vi "Teleop.vi"(10 "Match Info":T1={"Autonomous Elapsed Seconds"=0.0, "TeleOp Elapsed Seconds"=0.0, "Disabled Elapsed Seconds"=0.0, "Visited Autonomous"=FALSE, "Visited TeleOp"=FALSE, "Visited Disabled"=FALSE, "Autonomous Settings"={"Autonomous Style"=enum."Independent", "VI Refnum"=refnum}}, 11 "Call Context":T2) -> ()   [LabVIEW 2020]
doc: "This VI is called for each TeleOp packet received from the DS where the robot is not disabled. It is often used to read from the joysticks and update I/O or to update setpoints for timed control loops. It should complete and return within 20 milliseconds or it may miss DS packets."
uses:
  <vilib>/Rock Robotics/WPI/DriverStation/WPI_DriverStationDerivedRobotMode.ctl
  <vilib>/Rock Robotics/WPI/DriverStation/WPI_DriverStationMatch Info.ctl
  <vilib>/Rock Robotics/WPI/Solenoid/WPI_SolenoidValue.ctl
  <vilib>/Rock Robotics/WPI/ThirdParty/Phoenix-LabVIEW/Motor Controller/Controls/CTRE_Phoenix_MotorControl_ControlMode.ctl
  <vilib>/Rock Robotics/WPI/Utilities/WPI_GetSetVariantRefNum.vi
  <vilib>/Rock Robotics/Network Tables/NT Write Numeric Array.vi
  <vilib>/Rock Robotics/Network Tables/NT Read Boolean.vi
  <vilib>/Rock Robotics/Network Tables/NT Read Number.vi
  <vilib>/Rock Robotics/WPI/Solenoid/Deprecated/WPI_SolenoidSetBool.vi
  Robot Global Data.vi
  <vilib>/Rock Robotics/WPI/Solenoid/WPI_SolenoidSetEnum.vi
  <vilib>/Rock Robotics/Network Tables/NT Write Number.vi
  <vilib>/Rock Robotics/Network Tables/NT Write Boolean Array.vi
  <vilib>/Rock Robotics/WPI/Solenoid/Deprecated/WPI_SolenoidGetBool.vi
panel:
  out "TargetValid 5":bool
  out "TargetValid 4":bool
  out "POVs":i16[](array[numeric])
  out "Sample Slider 0":dbl(slide) scale=0.0..5.0
  out "Sample Boolean 1":bool
  out "Sample Boolean 0":bool
  # "April tags"
  # "Retroreflective tape"
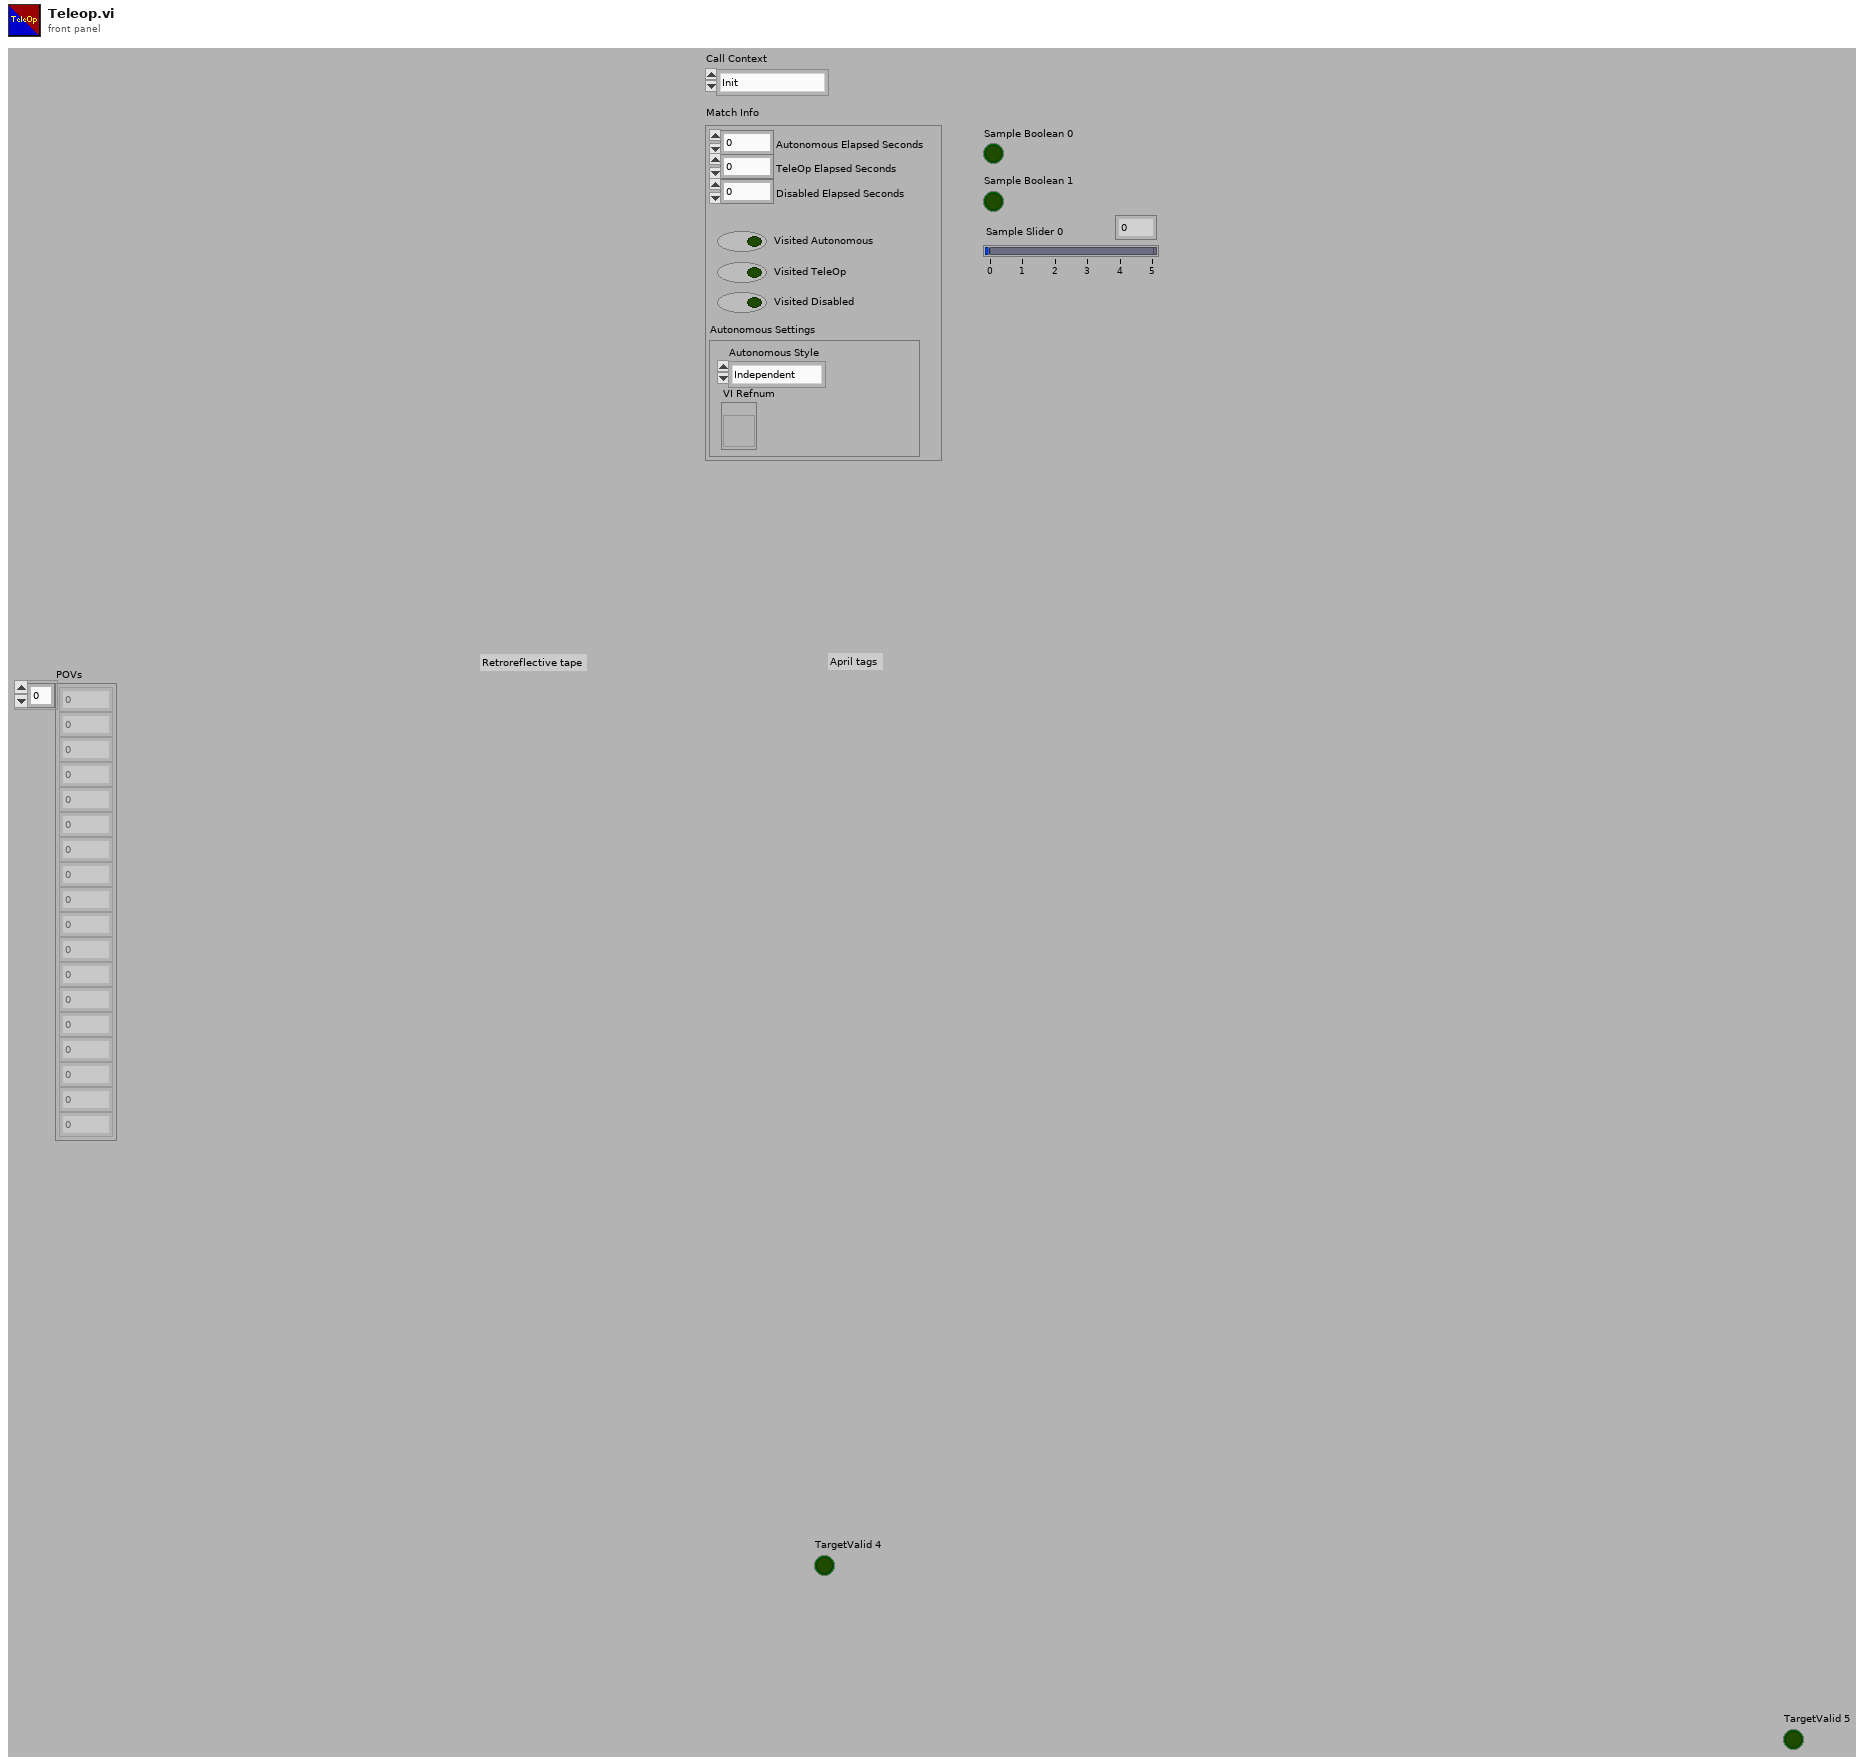
[diagram p1: front panel]
types:
  T1 = typedef "WPI_DriverStationMatch Info.ctl" = cluster{"Autonomous Elapsed Seconds":dbl, "TeleOp Elapsed Seconds":dbl, "Disabled Elapsed Seconds":dbl, "Visited Autonomous":bool, "Visited TeleOp":bool, "Visited Disabled":bool, "Autonomous Settings":cluster{"Autonomous Style":enum16{"Iterative", "Independent"}, "VI Refnum":refnum<vi>}}
  T2 = typedef "WPI_DriverStationDerivedRobotMode.ctl" = enum16{"Init", "Execute", "Stop"}
  T3 = typedef "WPI_SolenoidValue.ctl" = enum16{"Off", "On", "Forward", "Reverse"}
  T4 = cluster{"offsetAngle H":dbl, "offsetAngle V":dbl, "area":dbl, "skew":dbl}
  T5 = typedef "WPI_RobotDriveDevRef.ctl" = cluster{"DevStatus":errorcluster, "Motors[]":T6[], "Square Inputs":bool, "Max Output":dbl}
  T6 = typedef "WPI_MotorControlDeviceRef.ctl" = cluster{"DeviceStatus":errorcluster, "Type":T7, "PWM":cluster{"PWM Channel":T8, "DeadBand":T9}, "CAN":cluster{"Device Number":u8, "SetOutput VI Ref":variant, "GetOutput VI Ref":variant, "Enable VI Ref":variant, "Disable VI Ref":variant, "Data":variant}, "Invert":bool, "DIO PWM":cluster{"PWM \"Enable\" Channel":T8, "DIOChannel":T10, "PWM Rate":dbl}}
  T7 = typedef "WPI_MotorControlType.ctl" = enum16{"PWM", "CAN", "DIO PWM"}
  T8 = typedef "FPGA_DIOPWMChannel.ctl" = enum8{"PWM 0", "PWM 1", "PWM 2", "PWM 3", "PWM 4", "PWM 5", "PWM 6", "PWM 7", "PWM 8", "PWM 9", "PWM MXP 0", "PWM MXP 1", "PWM MXP 2", "PWM MXP 3", "PWM MXP 4", "PWM MXP 5", "PWM MXP 6", "PWM MXP 7", "PWM MXP 8", "PWM MXP 9", "Invalid"}
  T9 = typedef "WPI_PWMDeadband.ctl" = cluster{"Name":string, "maxPositivePwm":i32, "minPositivePwm":i32, "centerPwm":i32, "maxNegativePwm":i32, "minNegativePwm":i32, "angularRange":u16}
  T10 = typedef "FPGA_DIOChannel.ctl" = enum8{"DIO 0", "DIO 1", "DIO 2", "DIO 3", "DIO 4", "DIO 5", "DIO 6", "DIO 7", "DIO 8", "DIO 9", "DIO MXP 0", "DIO MXP 1", "DIO MXP 2", "DIO MXP 3", "DIO MXP 4", "DIO MXP 5", "DIO MXP 6", "DIO MXP 7", "DIO MXP 8", "DIO MXP 9", "DIO MXP 10", "DIO MXP 11", "DIO MXP 12", "DIO MXP 13", "DIO MXP 14", "DIO MXP 15", "SPI Port CS1", "SPI Port CS2", "SPI Port CS3", "SPI Port MISO", "SPI Port MOSI", "Invalid"}
  T11 = typedef "WPI_JoystickDevRef.ctl" = cluster{"Device":T12}
  T12 = typedef "WPI_JoystickDeviceEnum.ctl" = enum16{"USB 0", "USB 1", "USB 2", "USB 3", "USB 4", "USB 5"}
  T13 = cluster{"Buttons[0]":bool, "Buttons[1]":bool, "Buttons[2]":bool, "Buttons[3]":bool, "Buttons[4]":bool, "Buttons[5]":bool, "Buttons[6]":bool, "Buttons[7]":bool, "Buttons[8]":bool}
  T14 = cluster{"Axes[0]":dbl, "Axes[1]":dbl, "Axes[2]":dbl, "Axes[3]":dbl, "Axes[4]":dbl, "Axes[5]":dbl, "Axes[6]":dbl, "Axes[7]":dbl, "Axes[8]":dbl}
  T15 = typedef "WPI_SolenoidDevRef.ctl" = cluster{"DevStatus":errorcluster, "Pneumatics Control Module":u8, "Forward Solenoid Channel":T16, "Reverse Solenoid Channel":T16}
  T16 = typedef "WPI_SolenoidChannel.ctl" = enum8{"Solenoid 0", "Solenoid 1", "Solenoid 2", "Solenoid 3", "Solenoid 4", "Solenoid 5", "Solenoid 6", "Solenoid 7", "Solenoid 8", "Solenoid 9", "Solenoid 10", "Solenoid 11", "Solenoid 12", "Solenoid 13", "Solenoid 14", "Solenoid 15", "Invalid"}
  T17 = typedef "CTRE_Phoenix_MotorControl_ControlMode.ctl" = u16
  T18 = cluster{"Motors[][0]":T6, "Motors[][1]":T6, "Motors[][2]":T6, "Motors[][3]":T6, "Motors[][4]":T6, "Motors[][5]":T6, "Motors[][6]":T6, "Motors[][7]":T6, "Motors[][8]":T6}
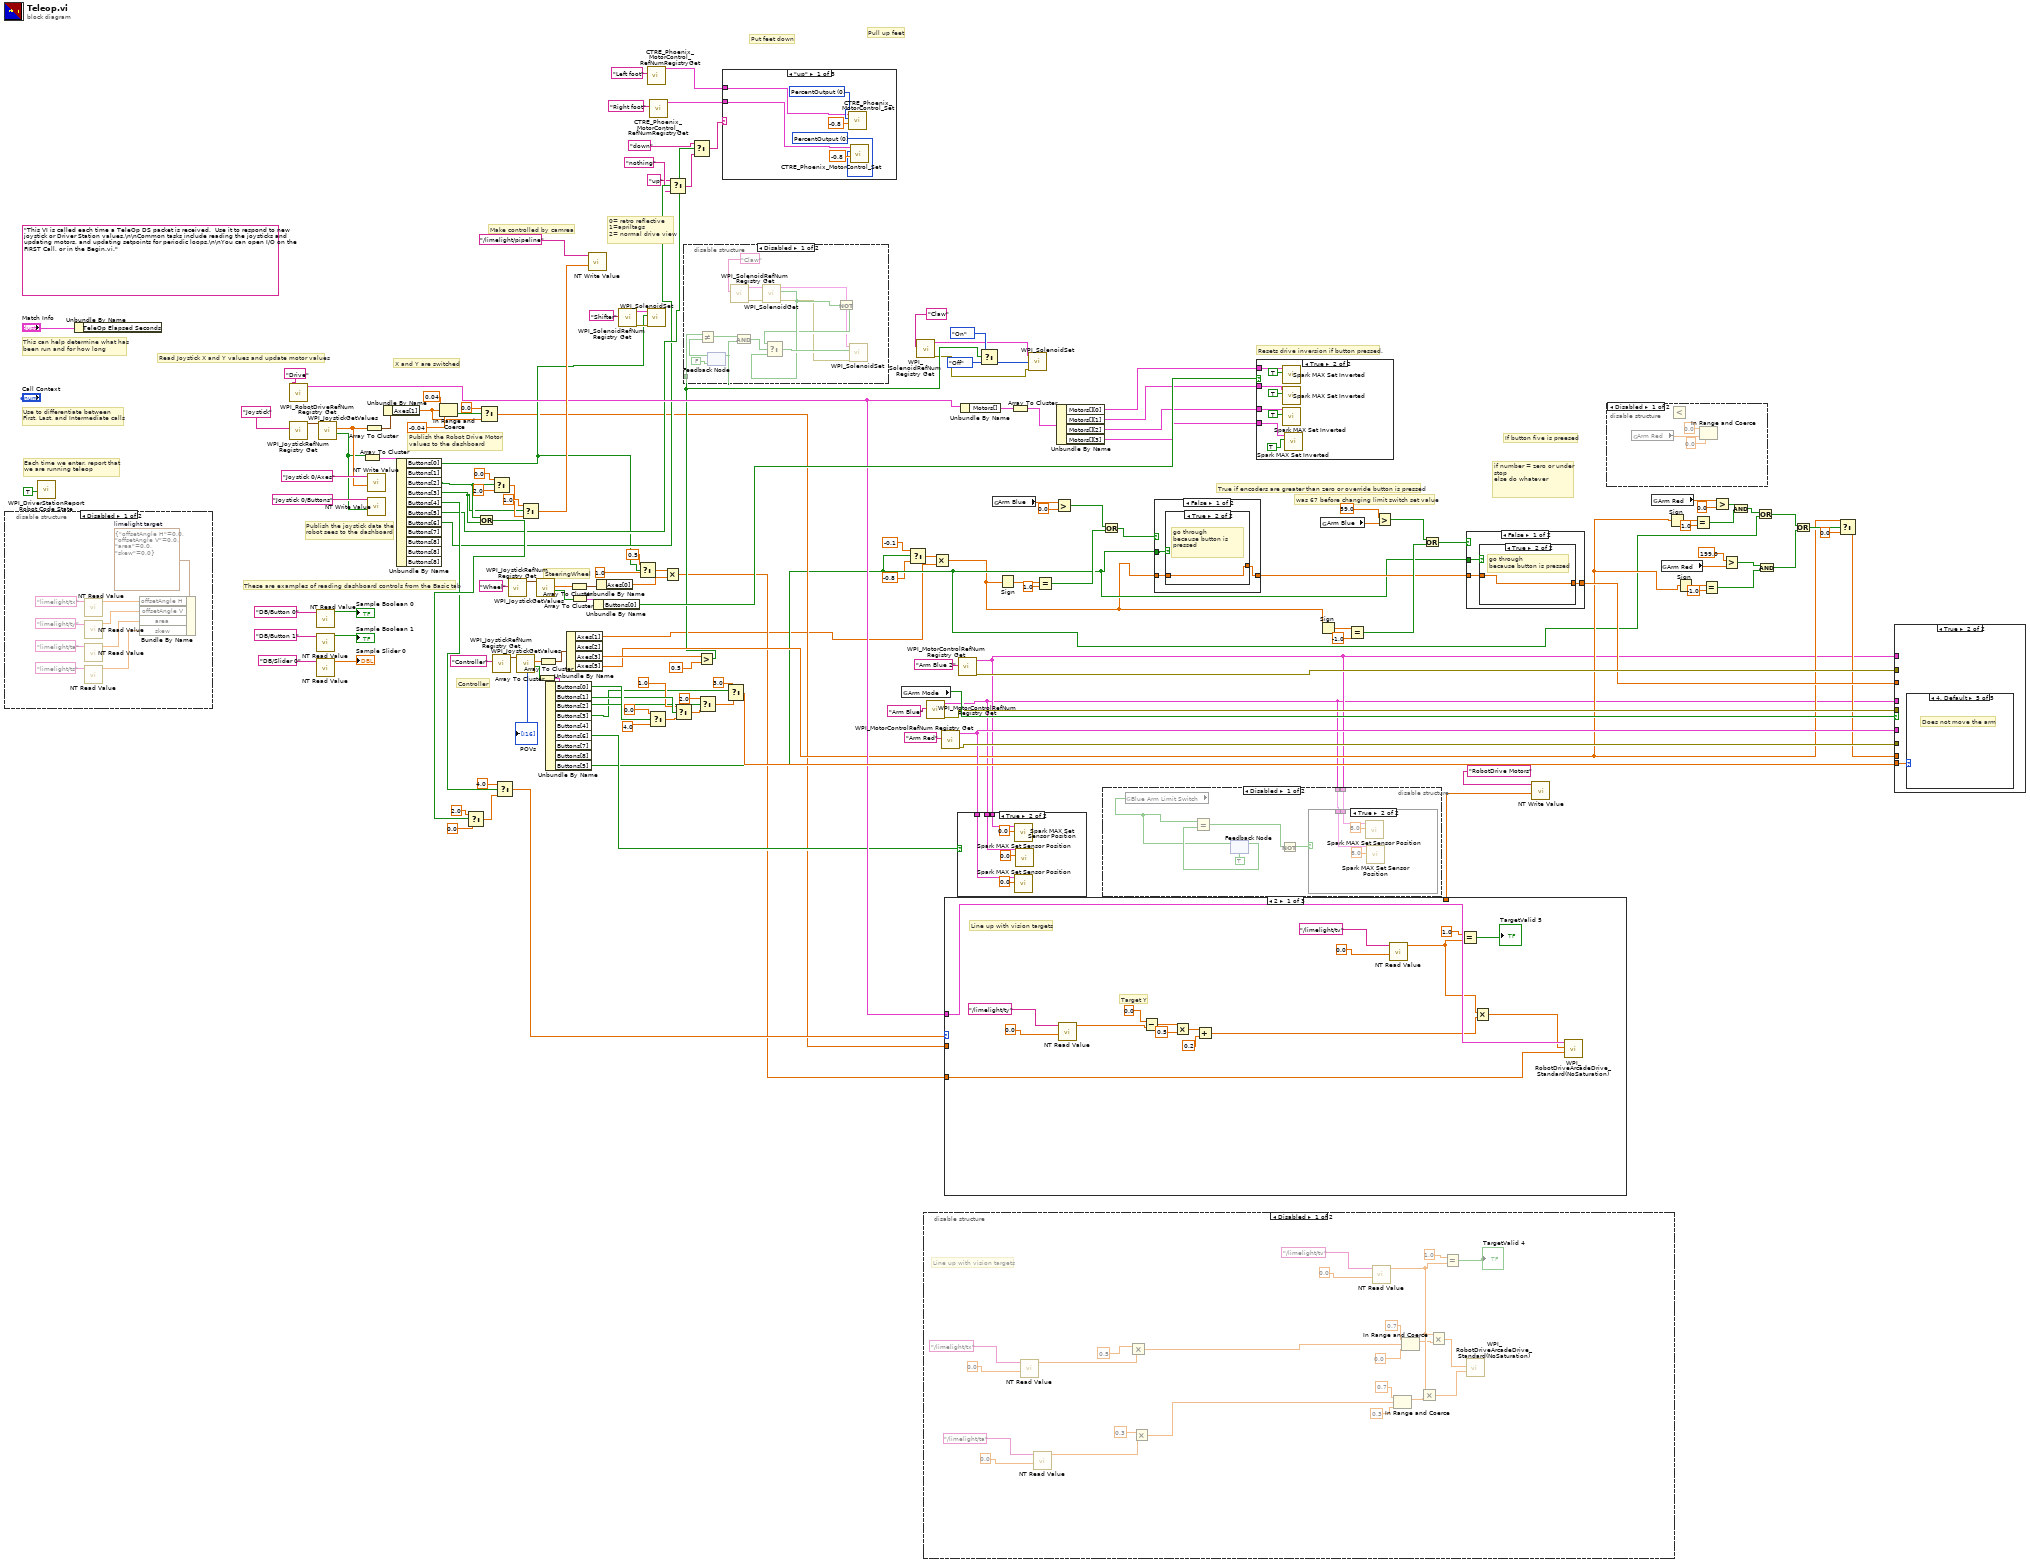
[diagram p0: block diagram]
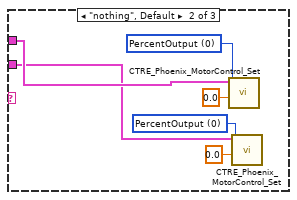
[diagram p6: hidden frame]
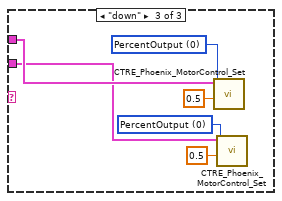
[diagram p7: hidden frame]
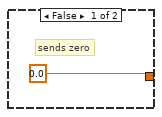
[diagram p8: hidden frame]
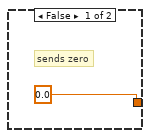
[diagram p10: hidden frame]
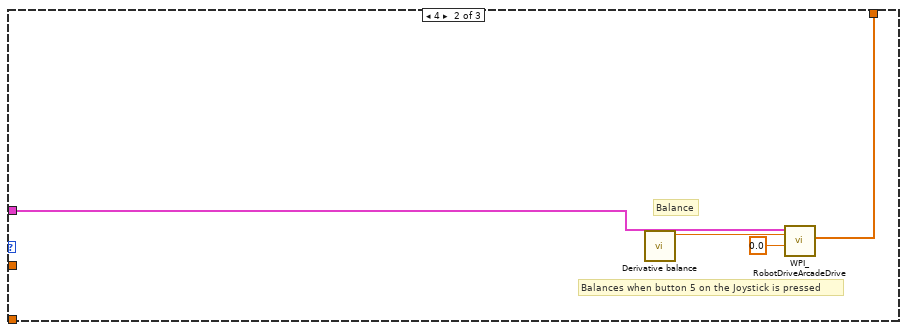
[diagram p15: hidden frame]
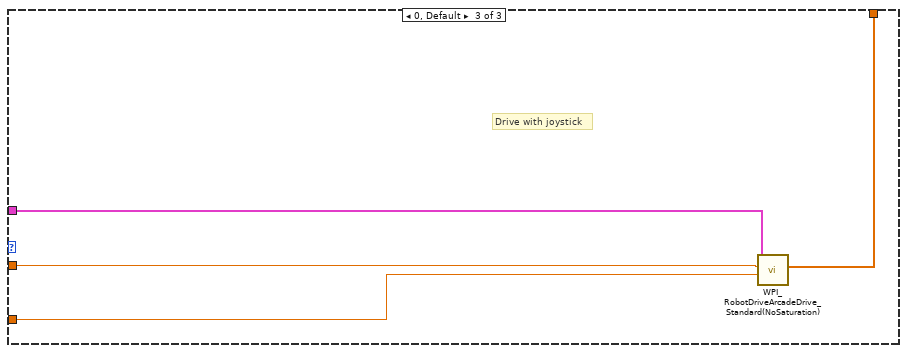
[diagram p16: hidden frame]
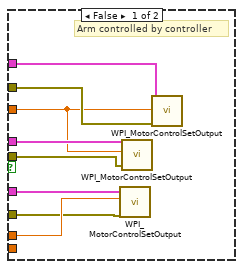
[diagram p17: hidden frame]
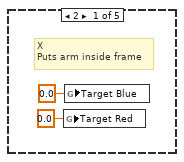
[diagram p18: hidden frame]
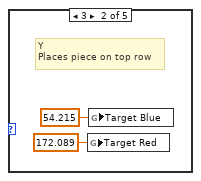
[diagram p19: hidden frame]
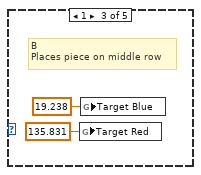
[diagram p20: hidden frame]
diagram:
  (unwired) "This VI is called each time a TeleOp DS packet is received.  Use it to respond to new joystick or Driver Station values.\n\nCommon tasks include reading the joysticks and updating motors, and updating setpoints for periodic loops.\n\nYou can open I/O on the FIRST Call, or in the Begin.vi."
  # "X and Y are switched"
  # "Put feet down"
  # "Pull up feet"
  # "was 67 before changing limit switch set value"
  # "True if encoders are greater than zero or override button is pressed"
  # "if number = zero or under\nstop\nelse do whatever"
  # "If button five is preesed"
  # "Resets drive inversion if button pressed."
  # "0= retro reflective\n1=apriltags\n2= normal drive view"
  # "Make controlled by camrea"
  # "SteeringWheel"
  # "Controller"
  # "These are examples of reading dashboard controls from the Basic tab"
  # "Publish the Robot Drive Motor\nvalues to the dashboard"
  # "Publish the joystick data the\nrobot sees to the dashboard"
  # "Each time we enter, report that\nwe are running teleop"
  # "Use to differentiate between\nFirst, Last, and Intermediate calls"
  # "This can help determine what has\nbeen run and for how long"
  # "Read Joystick X and Y values and update motor values"
  n1 = disable-structure shown="Disabled" {
    frame Disabled {
      w160 = T4 {"offsetAngle H"=0.0, "offsetAngle V"=0.0, "area"=0.0, "skew"=0.0}  # limelight target
      n2 = call-poly <vilib>:"NT Read Value.vi"("name"="limelight/tx" ("Name")) -> ("value"=w159:dbl)  [unwired: 8 in, 2 out]
      n3 = call-poly <vilib>:"NT Read Value.vi"("name"="limelight/ty" ("Name")) -> ("value"=w158:dbl)  [unwired: 8 in, 2 out]
      n4 = call-poly <vilib>:"NT Read Value.vi"("name"="limelight/ta" ("Name")) -> ("value"=w157:dbl)  [unwired: 8 in, 2 out]
      n5 = call-poly <vilib>:"NT Read Value.vi"("name"="limelight/ts" ("Name")) -> ("value"=w156:dbl)  [unwired: 8 in, 2 out]
      n6 = Bundle By Name(cluster=w160, "offsetAngle H"=w159, "offsetAngle V"=w158, "area"=w157, "skew"=w156) -> ()  [unwired: 1 out]
    }
    frame Enabled {
    }
  }
  n7 = call <vilib>:"WPI_DriverStationReport Robot Code State.vi"("TeleOp"=TRUE ("Autonomous")) -> ()  [unwired: 10 in, 1 out]
  n8 = Unbundle By Name("Match Info") -> ()  [unwired: 1 out]
  n9 = call <vilib>:"WPI_RobotDriveRefNum Registry Get.vi"("refnum name"="Drive") -> ("RobotDriveDevRef"=w80:T5)  [unwired: 1 in, 9 out]
  n10 = call <vilib>:"WPI_JoystickRefNum Registry Get.vi"("refnum name"="Joystick") -> ("JoystickDevRef"=w152:T11)  [unwired: 1 in, 9 out]
  n11 = call-poly <vilib>:"NT Read Value.vi"("name"="DB/Button 0" ("refnum name")) -> ("value"=→"Sample Boolean 0":bool)  [unwired: 8 in, 2 out]
  n12 = call-poly <vilib>:"NT Read Value.vi"("name"="DB/Slider 0" ("refnum name")) -> ("value"=→"Sample Slider 0":dbl)  [unwired: 8 in, 2 out]
  n13 = call-poly <vilib>:"NT Read Value.vi"("name"="DB/Button 1" ("refnum name")) -> ("value"=→"Sample Boolean 1":bool)  [unwired: 8 in, 2 out]
  n14 = call <vilib>:"WPI_JoystickGetValues.vi"("JoystickDevRef"=w152) -> ("Buttons"=w110:bool[], "Axes"=w141:dbl[])  [unwired: 6 in, 3 out]
  n15 = Array To Cluster(array=w110) -> (cluster=w109:T13)
  n16 = Array To Cluster(array=w141) -> (cluster=w140:T14)
  n17 = call-poly <vilib>:"NT Write Value.vi"("value"=w141, "name"="Joystick 0/Axes" ("Name")) -> ()  [unwired: 9 in, 1 out]
  n18 = call-poly <vilib>:"NT Write Value.vi"("value"=w110, "name"="Joystick 0/Buttons" ("Name")) -> ()  [unwired: 9 in, 1 out]
  n19 = Unbundle By Name(w140) -> ("Axes[1]"=w8:dbl)
  n20 = Unbundle By Name(w109) -> ("Buttons[0]"=w17:bool, "Buttons[2]"=w93:bool, "Buttons[3]"=w92:bool, "Buttons[4]"=w37:bool, "Buttons[5]"=w36:bool, "Buttons[6]"=w32:bool)  [unwired: 5 out]
  n21 = In Range and Coerce(upper limit=0.04, x=w8, lower limit=-0.04) -> (In Range?=w12:bool)  [unwired: 1 out]
  n22 = Or(x=w93, y=w92) -> (x .or. y?=w91:bool)
  n23 = Select(t=2.0, s=w91, f=0.0) -> (s? t:f=w106:dbl)
  n24 = Select(t=0.0, s=w12, f=w8) -> (s? t:f=w7:dbl)
  n25 = Select(t=0.0, s=w93, f=2.0) -> (s? t:f=w94:dbl)
  n26 = call <vilib>:"WPI_JoystickRefNum Registry Get.vi"("refnum name"="Controller") -> ("JoystickDevRef"=w134:T11)  [unwired: 9 in, 1 out]
  n27 = Select(t=4.0, s=w37, f=w106) -> (s? t:f=w104:dbl)
  n28 = call <vilib>:"WPI_JoystickRefNum Registry Get.vi"("refnum name"="Wheel") -> ("JoystickDevRef"=w138:T11)  [unwired: 9 in, 1 out]
  n29 = call <vilib>:"WPI_JoystickGetValues.vi"("JoystickDevRef"=w134) -> ("Buttons"=w131:bool[], "Axes"=w133:dbl[], "POVs"=→"POVs":i16[])  [unwired: 6 in, 2 out]
  n30 = Select(t=1.0, s=w92, f=w94) -> (s? t:f=w89:dbl)
  n31 = call <vilib>:"WPI_JoystickGetValues.vi"("JoystickDevRef"=w138) -> ("Buttons"=w85:bool[], "Axes"=w137:dbl[])  [unwired: 6 in, 3 out]
  n32 = Array To Cluster(array=w131) -> (cluster=w130:T13)
  n33 = Array To Cluster(array=w133) -> (cluster=w132:T14)
  n34 = Unbundle By Name(w130) -> ("Buttons[0]"=w128:bool, "Buttons[1]"=w123:bool, "Buttons[2]"=w116:bool, "Buttons[3]"=w115:bool, "Buttons[6]"=w38:bool, "Buttons[5]"=w6:bool)  [unwired: 3 out]
  n35 = Unbundle By Name(w132) -> ("Axes[1]"=w2:dbl, "Axes[3]"=w98:dbl, "Axes[5]"=w41:dbl)  [unwired: 1 out]
  n36 = Array To Cluster(array=w137) -> (cluster=w136:T14)
  n37 = Array To Cluster(array=w85) -> (cluster=w84:T13)
  n38 = call-poly <vilib>:"NT Write Value.vi"("value"=w89, "name"="/limelight/pipeline" ("Name")) -> ()  [unwired: 9 in, 1 out]
  n39 = Unbundle By Name(w84) -> ("Buttons[0]"=w83:bool)
  n40 = Unbundle By Name(w136) -> ("Axes[0]"=w16:dbl)
  n41 = call <vilib>:"WPI_SolenoidRefNum Registry Get.vi"("refnum name"="Shifter") -> ("error out"=w102:errorcluster, "SolenoidDevRef"=w101:T15)  [unwired: 9 in]
  n42 = Select(t=0.5, s=w17, f=1.0) -> (s? t:f=w18:dbl)
  n43 = call <vilib>:"CTRE_Phoenix_MotorControl_RefNumRegistryGet.vi"("refnum name"="Left foot") -> ("PhoenixMotorControlDevRef"=w26:T6)  [unwired: 9 in, 1 out]
  n44 = call-poly <vilib>:"WPI_SolenoidSet.vi"("error in (no error)"=w102, "Value"=w17, "SolenoidDevRef"=w101) -> ()  [unwired: 7 in, 2 out]
  n45 = call <vilib>:"CTRE_Phoenix_MotorControl_RefNumRegistryGet.vi"("refnum name"="Right foot") -> ("PhoenixMotorControlDevRef"=w27:T6)  [unwired: 9 in, 1 out]
  n46 = Select(t=0.0, s=w128, f=4.0) -> (s? t:f=w125:dbl)
  n47 = Multiply(x=w18, y=w16) -> (x*y=w15:dbl)
  n48 = Select(t="up", s=w32, f="nothing") -> (s? t:f=w33:string)
  n49 = Select(t=1.0, s=w123, f=w125) -> (s? t:f=w124:dbl)
  n50 = Select(t="down", s=w36, f=w33) -> (s? t:f=w34:string)
  n51 = Greater?(x=w98, y=0.5) -> (0:w21:bool)
  n52 = disable-structure shown="Disabled" {
    disable-tunnel: w21 -> [w172 _]
    frame Disabled {
      n53 = feedback #1(FALSE ("x > y?")) -> (w176:bool)
      n54 = Not Equal?(x=w172, y=w176) -> (x != y?=w174:bool)
      n55 = feedback-in #1(w172) -> ()
      n56 = call <vilib>:"WPI_SolenoidRefNum Registry Get.vi"("refnum name"="Claw") -> ("error out"=w170:errorcluster, "SolenoidDevRef"=w171:T15)  [unwired: 9 in]
      n57 = And(x=w174, y=w172) -> (x .and. y?=w173:bool)
      n58 = call-poly <vilib>:"WPI_SolenoidGet.vi"("error in (no error)"=w170, "SolenoidDevRef"=w171) -> ("error out"=w165:errorcluster, "Value"=w168:bool, "SolenoidDevRef"=w166:T15)  [unwired: 7 in]
      n59 = Not(x=w168) -> (.not. x?=w167:bool)
      n60 = Select(t=w167, s=w173, f=w168) -> (s? t:f=w177:bool)
      n61 = call-poly <vilib>:"WPI_SolenoidSet.vi"("error in (no error)"=w165, "Value"=w177, "SolenoidDevRef"=w166) -> ()  [unwired: 7 in, 2 out]
    }
    frame Enabled {
    }
  }
  n62 = Select(t=2.0, s=w116, f=w124) -> (s? t:f=w113:dbl)
  n63 = case shown="\"up\"" w34 {
    tunnel: w27 -> [w179 w184 w190]
    tunnel: w26 -> [w178 w185 w191]
    frame "up" {
      w182 = T17 0 items=["PercentOutput"=0, "Position"=1, "Velocity"=2, "Current"=3, "Follower"=5, "MotionProfile"=6, "MotionMagic"=7, "MotionProfileArc"=10, "Disabled"=15] ("Control Mode")
      w180 = T17 0 items=["PercentOutput"=0, "Position"=1, "Velocity"=2, "Current"=3, "Follower"=5, "MotionProfile"=6, "MotionMagic"=7, "MotionProfileArc"=10, "Disabled"=15] ("Control Mode")
      n64 = call <vilib>:"CTRE_Phoenix_MotorControl_Set.vi"("Output"=-0.8, "Control Mode"=w180, "PhoenixMotorControlDevRef"=w178) -> ()  [unwired: 7 in, 2 out]
      n65 = call <vilib>:"CTRE_Phoenix_MotorControl_Set.vi"("Output"=-0.8, "Control Mode"=w182, "PhoenixMotorControlDevRef"=w179) -> ()  [unwired: 7 in, 2 out]
    }
    frame "nothing", Default {
      w187 = T17 0 items=["PercentOutput"=0, "Position"=1, "Velocity"=2, "Current"=3, "Follower"=5, "MotionProfile"=6, "MotionMagic"=7, "MotionProfileArc"=10, "Disabled"=15] ("Control Mode")
      w189 = T17 0 items=["PercentOutput"=0, "Position"=1, "Velocity"=2, "Current"=3, "Follower"=5, "MotionProfile"=6, "MotionMagic"=7, "MotionProfileArc"=10, "Disabled"=15] ("Control Mode")
      n66 = call <vilib>:"CTRE_Phoenix_MotorControl_Set.vi"("Output"=0.0, "Control Mode"=w189, "PhoenixMotorControlDevRef"=w185) -> ()  [unwired: 7 in, 2 out]
      n67 = call <vilib>:"CTRE_Phoenix_MotorControl_Set.vi"("Output"=0.0, "Control Mode"=w187, "PhoenixMotorControlDevRef"=w184) -> ()  [unwired: 7 in, 2 out]
    }
    frame "down" {
      w193 = T17 0 items=["PercentOutput"=0, "Position"=1, "Velocity"=2, "Current"=3, "Follower"=5, "MotionProfile"=6, "MotionMagic"=7, "MotionProfileArc"=10, "Disabled"=15] ("Control Mode")
      w195 = T17 0 items=["PercentOutput"=0, "Position"=1, "Velocity"=2, "Current"=3, "Follower"=5, "MotionProfile"=6, "MotionMagic"=7, "MotionProfileArc"=10, "Disabled"=15] ("Control Mode")
      n68 = call <vilib>:"CTRE_Phoenix_MotorControl_Set.vi"("Output"=0.5, "Control Mode"=w195, "PhoenixMotorControlDevRef"=w191) -> ()  [unwired: 7 in, 2 out]
      n69 = call <vilib>:"CTRE_Phoenix_MotorControl_Set.vi"("Output"=0.5, "Control Mode"=w193, "PhoenixMotorControlDevRef"=w190) -> ()  [unwired: 7 in, 2 out]
    }
  }
  n70 = Select(t=3.0, s=w115, f=w113) -> (s? t:f=w112:dbl)
  n71 = global read "Robot Global Data.vi" "Arm Mode"() -> (w129:bool)
  n72 = Select(t=-0.1, s=w6, f=-0.8) -> (s? t:f=w5:dbl)
  n73 = call <vilib>:"WPI_SolenoidRefNum Registry Get.vi"("refnum name"="Claw") -> ("error out"=w19:errorcluster, "SolenoidDevRef"=w20:T15)  [unwired: 9 in]
  n74 = disable-structure shown="Disabled" {
    frame Disabled {
      # "Line up with vision targets"
      n75 = call-poly <vilib>:"NT Read Value.vi"("default value"=0.0 ("Default Value"), "name"="/limelight/tx" ("Name")) -> ("value"=w197:dbl)  [unwired: 7 in, 2 out]
      n76 = call-poly <vilib>:"NT Read Value.vi"("default value"=0.0 ("Default Value"), "name"="/limelight/ta" ("Name")) -> ("value"=w201:dbl)  [unwired: 7 in, 2 out]
      n77 = Multiply(x=0.5, y=w197) -> (x*y=w196:dbl)
      n78 = Multiply(x=0.3, y=w201) -> (x*y=w200:dbl)
      n79 = call-poly <vilib>:"NT Read Value.vi"("default value"=0.0 ("Default Value"), "name"="/limelight/tv" ("Name")) -> ("value"=w208:dbl)  [unwired: 7 in, 2 out]
      n80 = In Range and Coerce(upper limit=0.7, x=w200, lower limit=0.3) -> (coerced(x)=w207:dbl)  [unwired: 1 out]
      n81 = In Range and Coerce(upper limit=0.7, x=w196, lower limit=0.0) -> (coerced(x)=w206:dbl)  [unwired: 1 out]
      n82 = Multiply(x=w208, y=w207) -> (x*y=w210:dbl)
      n83 = Multiply(x=w208, y=w206) -> (x*y=w209:dbl)
      n84 = Equal?(x=1.0, y=w208) -> (x = y?=→"TargetValid 4":bool)
      n85 = call <vilib>:"WPI_RobotDriveArcadeDrive_Standard(NoSaturation).vi"("Y axis value"=w210, "X axis value"=w209) -> ()  [unwired: 2 in, 8 out]
    }
    frame Enabled {
    }
  }
  n86 = call <vilib>:"WPI_MotorControlRefNum Registry Get.vi"("refnum name"="Arm Blue") -> ("error out"=w119:errorcluster, "MotorControlDevRef"=w39:T6)  [unwired: 9 in]
  n87 = Multiply(x=w5, y=w2) -> (x*y=w1:dbl)
  n88 = call <vilib>:"WPI_MotorControlRefNum Registry Get.vi"("refnum name"="Arm Red") -> ("error out"=w117:errorcluster, "MotorControlDevRef"=w86:T6)  [unwired: 9 in]
  n89 = case shown="2" w104 {
    tunnel: w80 -> [w233 w239 w243]
    tunnel: w7 -> [_ _ w242]
    tunnel: w15 -> [w219 _ w241]
    tunnel: [_ w238 w240] -> w103
    frame 2 {
      # "Target Y"
      # "Line up with vision targets"
      n90 = call-poly <vilib>:"NT Read Value.vi"("default value"=0.0 ("Default Value"), "name"="/limelight/ty" ("Name")) -> ("value"=w223:dbl)  [unwired: 7 in, 2 out]
      n91 = Subtract(x=0.0, y=w223) -> (x-y=w232:dbl)
      n92 = Multiply(x=w232, y=0.5) -> (x*y=w224:dbl)
      n93 = Add(x=w224, y=0.2) -> (x+y=w220:dbl)
      n94 = call-poly <vilib>:"NT Read Value.vi"("default value"=0.0 ("Default Value"), "name"="/limelight/tv" ("Name")) -> ("value"=w227:dbl)  [unwired: 7 in, 2 out]
      n95 = Equal?(x=1.0, y=w227) -> (x = y?=→"TargetValid 5":bool)
      n96 = Multiply(x=w227, y=w220) -> (x*y=w226:dbl)
      n97 = call <vilib>:"WPI_RobotDriveArcadeDrive_Standard(NoSaturation).vi"("Y axis value"=w219, "X axis value"=w226, "RobotDriveDevRef"=w233) -> ()  [unwired: 1 in, 8 out]
    }
    frame 4 {
      # "Balances when button 5 on the Joystick is pressed"
      # "Balance"
      n98 = call "Derivative balance.vi"() -> ("Motor Power"=w237:dbl)  [unwired: 11 in]
      n99 = call-poly <vilib>:"WPI_RobotDriveArcadeDrive.vi"("Y axis value"=0.0, "X axis value"=w237, "RobotDriveDevRef"=w239) -> ("Motor Values"=w238:dbl[])  [unwired: 6 in, 2 out]
    }
    frame 0, Default {
      # "Drive with joystick"
      n100 = call <vilib>:"WPI_RobotDriveArcadeDrive_Standard(NoSaturation).vi"("Y axis value"=w241, "X axis value"=w242, "RobotDriveDevRef"=w243) -> ("Motor Values"=w240:dbl[])  [unwired: 1 in, 7 out]
    }
  }
  n101 = call <vilib>:"WPI_MotorControlRefNum Registry Get.vi"("refnum name"="Arm Blue 2") -> ("error out"=w87:errorcluster, "MotorControlDevRef"=w40:T6)  [unwired: 9 in]
  n102 = case shown="True" w38 {
    tunnel: w40 -> [_ w249]
    tunnel: w39 -> [_ w248]
    tunnel: w86 -> [_ w247]
    frame False {
    }
    frame True {
      n103 = call <vilib>:"Spark MAX Set Sensor Position.vi"("Position"=0.0, "MotorControlDeviceRef"=w249) -> ()  [unwired: 8 in, 2 out]
      n104 = call <vilib>:"Spark MAX Set Sensor Position.vi"("Position"=0.0, "MotorControlDeviceRef"=w247) -> ()  [unwired: 8 in, 2 out]
      n105 = call <vilib>:"Spark MAX Set Sensor Position.vi"("Position"=0.0, "MotorControlDeviceRef"=w248) -> ()  [unwired: 8 in, 2 out]
    }
  }
  n106 = Unbundle By Name(w80) -> ("Motors[]"=w82:T6[])
  n107 = Select(t=WPI_SolenoidValue."On" ("Value"), s=w21, f=WPI_SolenoidValue."Off" ("Value")) -> (s? t:f=w24:T3)
  n108 = global read "Robot Global Data.vi" "Arm Blue"() -> (w75:dbl)
  n109 = Sign(1:w1) -> (0:w72:dbl)
  n110 = Array To Cluster(array=w82) -> (cluster=w81:T18)
  n111 = call-poly <vilib>:"WPI_SolenoidSet.vi"("error in (no error)"=w19, "Value"=w24, "SolenoidDevRef"=w20) -> ()  [unwired: 7 in, 2 out]
  n112 = Equal?(x=w72, y=1.0) -> (x = y?=w70:bool)
  n113 = Greater?(x=w75, y=0.0) -> (0:w74:bool)
  n114 = Unbundle By Name(w81) -> ("Motors[][0]"=w79:T6, "Motors[][1]"=w77:T6, "Motors[][2]"=w76:T6, "Motors[][3]"=w78:T6)
  n115 = Or(x=w74, y=w70) -> (x .or. y?=w69:bool)
  n116 = disable-structure shown="Disabled" {
    disable-tunnel: w40 -> [w255 _]
    disable-tunnel: w39 -> [w254 _]
    frame Disabled {
      n117 = global read "Robot Global Data.vi" "Blue Arm Limit Switch"() -> (w251:bool)
      n118 = feedback #2(TRUE) -> (w252:bool)
      n119 = Equal?(x=w251, y=w252) -> (x = y?=w250:bool)
      n120 = feedback-in #2(w251) -> ()
      n121 = Not(x=w250) -> (.not. x?=w256:bool)
      n122 = case shown="True" w256 {
        tunnel: w255 -> [_ w260]
        tunnel: w254 -> [_ w259]
        frame False {
        }
        frame True {
          n123 = call <vilib>:"Spark MAX Set Sensor Position.vi"("Position"=8.0, "MotorControlDeviceRef"=w260) -> ()  [unwired: 8 in, 2 out]
          n124 = call <vilib>:"Spark MAX Set Sensor Position.vi"("Position"=8.0, "MotorControlDeviceRef"=w259) -> ()  [unwired: 8 in, 2 out]
        }
      }
    }
    frame Enabled {
    }
  }
  n125 = case shown="False" w69 {
    tunnel: w6 -> [w263 _]
    tunnel: [w262 w266] -> w61
    tunnel: w1 -> [w261 w266]
    frame False {
      n126 = case shown="True" w263 {
        tunnel: [0.0 w265] -> w262
        tunnel: w261 -> [_ w265]
        frame False {
          # "sends zero"
        }
        frame True {
          # "go through\nbecause button is pressed"
        }
      }
    }
    frame True {
      # "go through if\nin range or moveing in right derection"
    }
  }
  n127 = case shown="True" w83 {
    tunnel: w79 -> [_ w274]
    tunnel: w78 -> [_ w269]
    tunnel: w77 -> [_ w268]
    tunnel: w76 -> [_ w267]
    frame False {
    }
    frame True {
      n128 = call <vilib>:"Spark MAX Set Inverted.vi"("Inverted (F)"=TRUE, "MotorControlDeviceRef in"=w274) -> ()  [unwired: 8 in, 2 out]
      n129 = call <vilib>:"Spark MAX Set Inverted.vi"("Inverted (F)"=TRUE, "MotorControlDeviceRef in"=w268) -> ()  [unwired: 8 in, 2 out]
      n130 = call <vilib>:"Spark MAX Set Inverted.vi"("Inverted (F)"=TRUE, "MotorControlDeviceRef in"=w267) -> ()  [unwired: 8 in, 2 out]
      n131 = call <vilib>:"Spark MAX Set Inverted.vi"("Inverted (F)"=TRUE, "MotorControlDeviceRef in"=w269) -> ()  [unwired: 8 in, 2 out]
    }
  }
  n132 = Sign(1:w1) -> (0:w67:dbl)
  n133 = global read "Robot Global Data.vi" "Arm Blue"() -> (w63:dbl)
  n134 = Equal?(x=w67, y=-1.0) -> (x = y?=w65:bool)
  n135 = Greater?(x=59.0 ("y"), y=w63) -> (0:w68:bool)
  n136 = Or(x=w68, y=w65) -> (x .or. y?=w64:bool)
  n137 = case shown="False" w64 {
    tunnel: w6 -> [w277 _]
    tunnel: [w276 w280] -> w60
    tunnel: w61 -> [w275 w280]
    frame False {
      n138 = case shown="True" w277 {
        tunnel: [0.0 w279] -> w276
        tunnel: w275 -> [_ w279]
        frame False {
          # "sends zero"
        }
        frame True {
          # "go through\nbecause button is pressed"
        }
      }
    }
    frame True {
      # "go through if\nin range or moveing in right derection"
    }
  }
  n139 = call-poly <vilib>:"NT Write Value.vi"("value"=w103, "name"="RobotDrive Motors" ("Name")) -> ()  [unwired: 9 in, 1 out]
  n140 = disable-structure shown="Disabled" {
    frame Disabled {
      n141 = global read "Robot Global Data.vi" "Arm Red"() -> (w281:dbl)
      n142 = Less?() -> ()  [unwired: 2 in, 1 out]
      n143 = In Range and Coerce(upper limit=0.0, x=w281, lower limit=0.0) -> ()  [unwired: 2 out]
    }
    frame Enabled {
    }
  }
  n144 = global read "Robot Global Data.vi" "Arm Red"() -> (w59:dbl)
  n145 = global read "Robot Global Data.vi" "Arm Red"() -> (w53:dbl)
  n146 = Sign(1:w41) -> (0:w57:dbl)
  n147 = Sign(1:w41) -> (0:w55:dbl)
  n148 = Equal?(x=w57, y=1.0) -> (x = y?=w50:bool)
  n149 = Equal?(x=w55, y=-1.0) -> (x = y?=w49:bool)
  n150 = Greater?(x=w59, y=0.0) -> (0:w51:bool)
  n151 = Greater?(x=199.0 ("y"), y=w53) -> (0:w48:bool)
  n152 = And(x=w51, y=w50) -> (x .and. y?=w47:bool)
  n153 = Or(x=w47, y=w6) -> (x .or. y?=w45:bool)
  n154 = And(x=w48, y=w49) -> (x .and. y?=w46:bool)
  n155 = Or(x=w45, y=w46) -> (x .or. y?=w44:bool)
  n156 = Select(t=w41, s=w44, f=0.0) -> (s? t:f=w42:dbl)
  n157 = case shown="True" w129 {
    tunnel: w42 -> [w291 _]
    tunnel: w119 -> [w290 _]
    tunnel: w39 -> [w289 _]
    tunnel: w117 -> [w288 _]
    tunnel: w86 -> [w287 _]
    tunnel: w112 -> [_ w292]
    tunnel: w40 -> [w286 _]
    tunnel: w87 -> [w285 _]
    tunnel: w60 -> [w284 _]
    frame False {
      # "Arm controlled by controller"
      n158 = call <vilib>:"WPI_MotorControlSetOutput.vi"("error in (no error)"=w288, "Output"=w291, "MotorControlDevRef"=w287) -> ()  [unwired: 6 in, 3 out]
      n159 = call <vilib>:"WPI_MotorControlSetOutput.vi"("error in (no error)"=w290, "Output"=w284, "MotorControlDevRef"=w289) -> ()  [unwired: 6 in, 3 out]
      n160 = call <vilib>:"WPI_MotorControlSetOutput.vi"("error in (no error)"=w285, "Output"=w284, "MotorControlDevRef"=w286) -> ()  [unwired: 6 in, 3 out]
    }
    frame True {
      n161 = case shown="4, Default" w292 {
        frame 2 {
          # "X\nPuts arm inside frame"
          n162 = global write "Robot Global Data.vi" "Target Red"(0.0 ("Target Red")) -> ()
          n163 = global write "Robot Global Data.vi" "Target Blue"(0.0 ("Target Blue")) -> ()
        }
        frame 3 {
          # "Y\nPlaces piece on top row"
          n164 = global write "Robot Global Data.vi" "Target Red"(172.089 ("Target Red")) -> ()
          n165 = global write "Robot Global Data.vi" "Target Blue"(54.215 ("Target Blue")) -> ()
        }
        frame 1 {
          # "B\nPlaces piece on middle row"
          n166 = global write "Robot Global Data.vi" "Target Red"(135.831 ("Target Red")) -> ()
          n167 = global write "Robot Global Data.vi" "Target Blue"(19.238 ("Target Blue")) -> ()
        }
        frame 0 {
          # "A\nPlaces piece on bottom row"
          n168 = global write "Robot Global Data.vi" "Target Red"(34.7616 ("Target Red")) -> ()
          n169 = global write "Robot Global Data.vi" "Target Blue"(33.3568 ("Target Blue")) -> ()
        }
        frame 4, Default {
          # "Does not move the arm"
        }
      }
    }
  }
